vi "PWM lenkberechnung.vi"(0 "wert vorne":dbl, 1 "gewicht vorne":dbl, 2 "wert schräg":dbl, 3 "gewicht schräg":dbl, 4 "wert seiten":dbl, 5 "gewicht seiten":dbl) -> (16 "ausgabe zu pide":dbl)   [LabVIEW 2016]
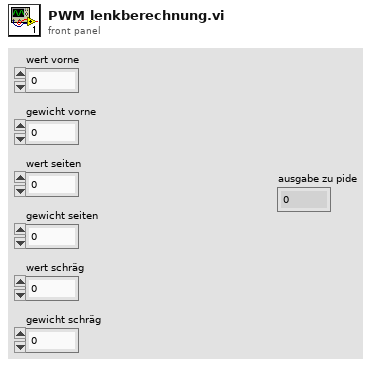
[diagram p1: front panel]
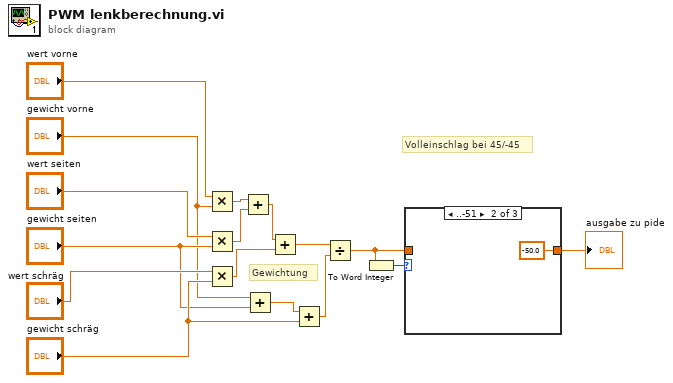
[diagram p0: block diagram]
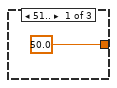
[diagram p2: hidden frame]
diagram:
  # "Volleinschlag bei 45/-45"
  # "Gewichtung"
  n1 = Multiply(x="wert vorne", y="gewicht vorne") -> (x*y=w14:dbl)
  n2 = Multiply(x="wert seiten", y="gewicht seiten") -> (x*y=w6:dbl)
  n3 = Multiply(x="wert schräg", y="gewicht schräg") -> (x*y=w9:dbl)
  n4 = Add(x=w14, y=w6) -> (x+y=w13:dbl)
  n5 = Add(x="gewicht vorne", y="gewicht seiten") -> (x+y=w11:dbl)
  n6 = Add(x=w13, y=w9) -> (x+y=w12:dbl)
  n7 = Add(x=w11, y="gewicht schräg") -> (x+y=w10:dbl)
  n8 = Divide(x=w12, y=w10) -> (x/y=w15:dbl)
  n9 = To Word Integer(number=w15) -> (16bit integer=w16:i16)
  n10 = case shown="..-51" w16 {
    tunnel: w15 -> [_ _ w19]
    tunnel: [50.0 -50.0 w19] -> w8
    frame 51.. {
    }
    frame ..-51 {
    }
    frame -50..50 {
    }
  }
  "ausgabe zu pide" <- w8
